vi "UI - Initiate Connection - Copy.vi"(8 "error in (no error)":errorcluster, 10 "Controller Address":string, 11 "Message Queue":refnum<queue>) -> (0 "error out":errorcluster, 1 "Connected?":bool)   [LabVIEW 2017]
uses:
  Message Queue/Message Cluster.ctl
  controls/FPGA State.ctl
  controls/CPU Loads.ctl
  Globals/Global - Configuration Options.vi
  Globals/Global - UI Stream and Variable Connections.vi
  Message Queue/Message Queue.lvlib
panel:
  out "error out 2":errorcluster
  out "tag acc":refnum<k21>
  out "Tag acc":refnum<k21>
  out "Variable Name Control/Indicator 2":refnum<k21>
  out "Variable Name Control/Indicator":refnum<k21>
  out "resulting string 2":string
  out "reader name":string="UI Reader"
  out "writer name":string="UI Writer"
  out "resulting string":string
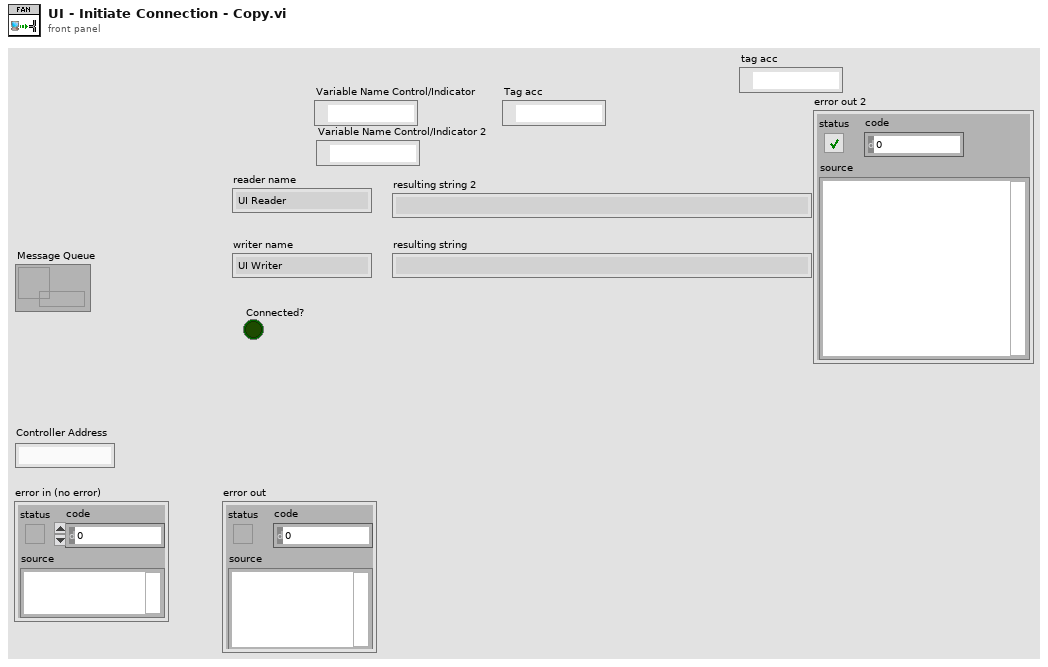
[diagram p1: front panel]
types:
  T1 = typedef "CPU Loads.ctl" = cluster{"Total (%)":dbl, "Time Critical (%)":dbl, "Timed Structures (%)":dbl, "High (%)":dbl, "Above Normal (%)":dbl, "Normal (%)":dbl, "Background (%)":dbl, "Idle (%)":dbl, "ISR (%)":dbl}[]
  T2 = typedef "FPGA State.ctl" = enum16{"Safe State", "Control (PID)"}
  T3 = typedef "Message Queue.lvlib/Message Cluster.ctl" = cluster{"Message":string, "Message Data":variant}
  T4 = cluster{"Actual PID Loop Period":refnum<k21>, "DMA FIFO Overflow?":refnum<k21>, "CPU Usage":refnum<k21>, "Free or Contiguous Memory":refnum<k21>, "Current FPGA State":refnum<k21>, "Acceleration (grms)":refnum<k21>, "Acceleration Waveform":refnum<k21>, "Chatter":refnum<k21>, "tag acc":refnum<k21>, "tag video":refnum<k21>}
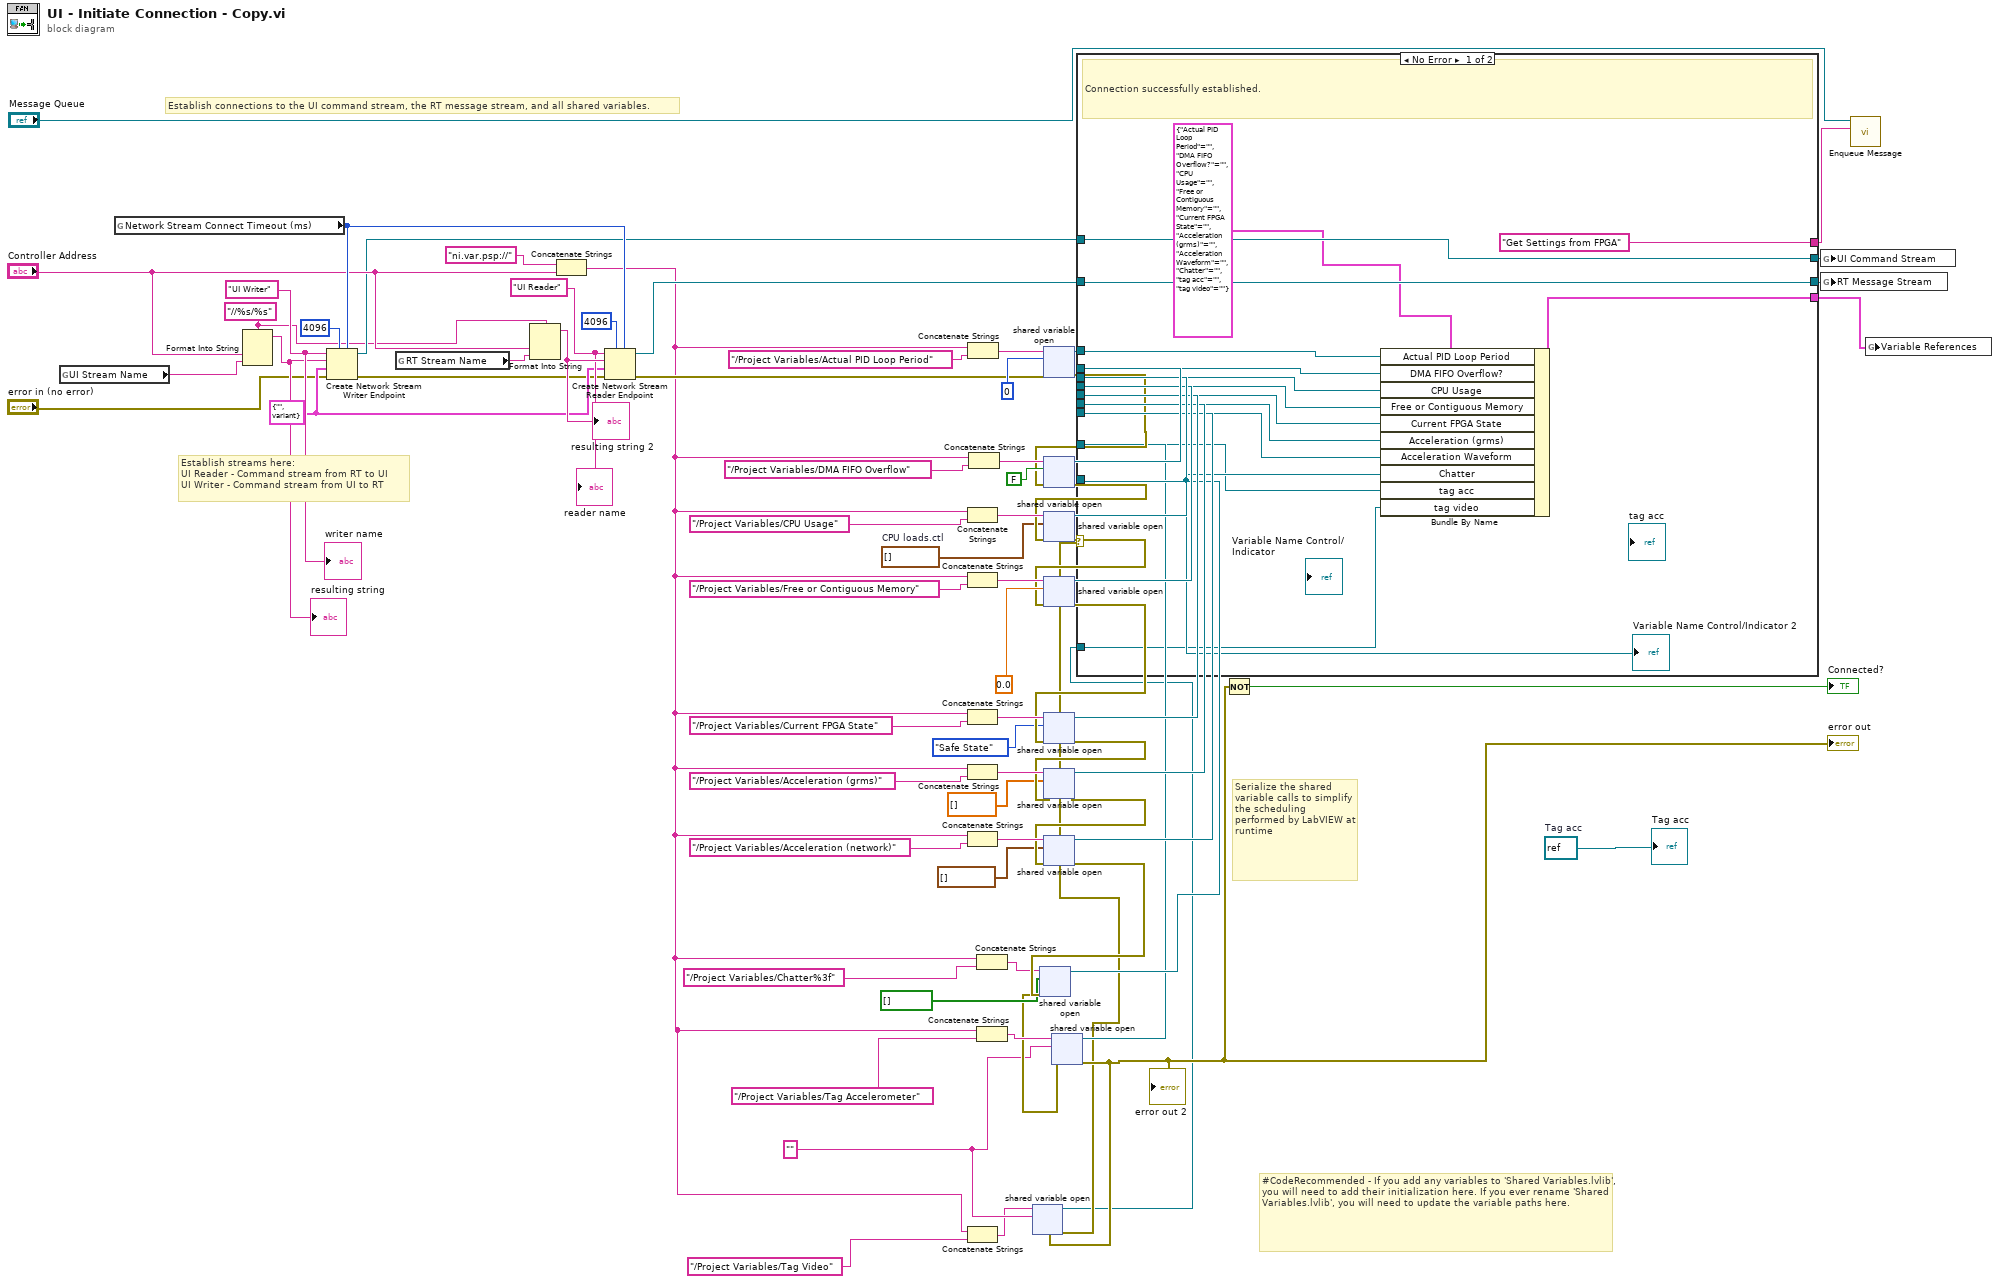
[diagram p0: block diagram]
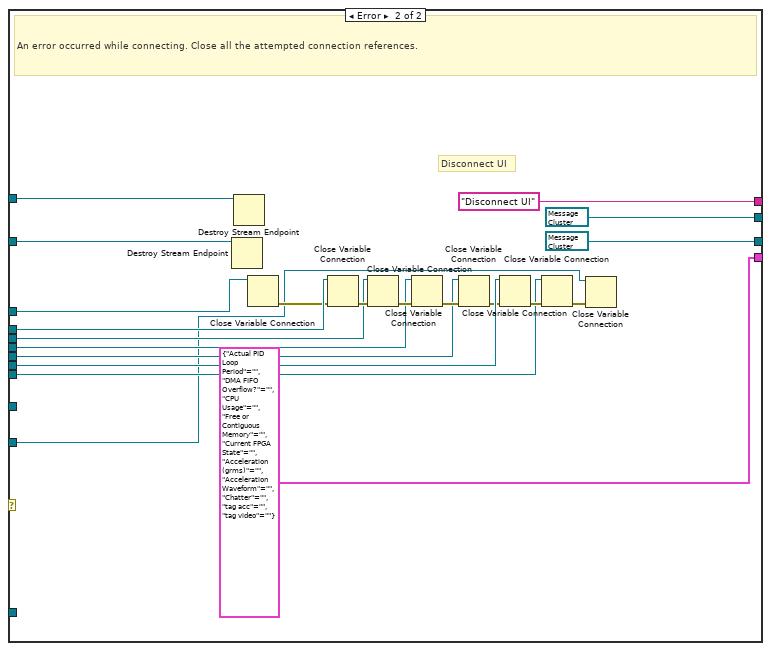
[diagram p2: hidden frame]
diagram:
  w5 = "" ("string")
  w9 = refnum<k21> refnum  # Tag acc
  w24 = T1 []  # CPU loads.ctl
  w70 = T3 {"Message"="", "Message Data"=variant} ("Message Cluster")
  w71 = "UI Reader" ("reader name")
  w74 = "UI Writer" ("writer name")
  w16 = "//%s/%s"
  # "Establish connections to the UI command stream, the RT message stream, and all shared variables."
  # "#CodeRecommended - If you add any variables to 'Shared Variables.lvlib', you will need to add their initialization here. If you ever rename 'Shared Variables.lvlib', you will need to update the variable paths here."
  # "Establish streams here:\nUI Reader - Command stream from RT to UI\nUI Writer - Command stream from UI to RT"
  # "Serialize the shared variable calls to simplify the scheduling performed by LabVIEW at runtime"
  n1 = global read "Global - Configuration Options.vi" "UI Stream Name"() -> (w15:string)
  n2 = global read "Global - Configuration Options.vi" "Network Stream Connect Timeout (ms)"() -> (w69:i32)
  n3 = Format Into String(format string=w16, "Controller Address", w15) -> (resulting string=w73:string)  [unwired: 2 in, 1 out]
  "resulting string" <- w73
  n4 = Create Network Stream Writer Endpoint(5:w69, 7:4096 ("writer buffer size"), 8:"error in (no error)", 9:w70, 10:w73, 11:w74) -> (0:w48:errorcluster, 3:w55:refnum<k21>)  [unwired: 1 in]
  n5 = global read "Global - Configuration Options.vi" "RT Stream Name"() -> (w14:string)
  n6 = Format Into String(format string=w16, "Controller Address", w14) -> (resulting string=w72:string)  [unwired: 2 in, 1 out]
  "resulting string 2" <- w72
  n7 = Concatenate Strings("ni.var.psp://", "Controller Address") -> (w6:string)
  n8 = Create Network Stream Reader Endpoint(5:w69, 7:4096 ("reader buffer size"), 8:w48, 9:w70, 10:w72, 11:w71) -> (0:w47:errorcluster, 3:w54:refnum<k21>)  [unwired: 1 in]
  n9 = Concatenate Strings(w6, "/Project Variables/CPU Usage") -> (w60:string)
  n10 = Concatenate Strings(w6, "/Project Variables/Free or Contiguous Memory") -> (w43:string)
  n11 = Concatenate Strings(w6, "/Project Variables/Current FPGA State") -> (w40:string)
  n12 = Concatenate Strings(w6, "/Project Variables/Acceleration (grms)") -> (w39:string)
  n13 = Concatenate Strings(w6, "/Project Variables/Acceleration (network)") -> (w36:string)
  n14 = Concatenate Strings(w6, "/Project Variables/Tag Video") -> (w1:string)
  n15 = Concatenate Strings(w6, "/Project Variables/Actual PID Loop Period") -> (w65:string)
  n16 = Concatenate Strings(w6, "/Project Variables/DMA FIFO Overflow") -> (w63:string)
  n17 = Concatenate Strings(w6, "/Project Variables/Chatter%3f") -> (w19:string)
  n18 = Concatenate Strings(w6, "/Project Variables/Tag Accelerometer") -> (w13:string)
  n19 = shared-variable-open(w65, w47, u32 0) -> (w58:refnum<k21>, w17:errorcluster)  [unwired: 1 in]
  n20 = shared-variable-open(w63, w17, FALSE ("data type")) -> (w57:refnum<k21>, w59:errorcluster)  [unwired: 1 in]
  n21 = shared-variable-open(w60, w59, w24) -> (w56:refnum<k21>, w35:errorcluster)  [unwired: 1 in]
  n22 = shared-variable-open(w43, w35, 0.0) -> (w30:refnum<k21>, w34:errorcluster)  [unwired: 1 in]
  n23 = shared-variable-open(w40, w34, FPGA_State."Safe State" ("FPGA State")) -> (w29:refnum<k21>, w33:errorcluster)  [unwired: 1 in]
  n24 = shared-variable-open(w39, w33, dbl[] []) -> (w28:refnum<k21>, w32:errorcluster)  [unwired: 1 in]
  n25 = shared-variable-open(w36, w32, waveform(dbl)[] []) -> (w27:refnum<k21>, w21:errorcluster)  [unwired: 1 in]
  n26 = shared-variable-open(w19, w21, bool[] []) -> (w18:refnum<k21>, w10:errorcluster)  [unwired: 1 in]
  n27 = shared-variable-open(w13, w10, w5) -> (w11:refnum<k21>, w4:errorcluster)  [unwired: 1 in]
  "error out" <- w4
  "error out 2" <- w4
  n28 = shared-variable-open(w1, w4, w5) -> (w2:refnum<k21>, w3:errorcluster)  [unwired: 1 in]
  n29 = case shown="No Error" w3 {
    tunnel: w58 -> [w90 w108]
    tunnel: w57 -> [w86 w106]
    tunnel: w56 -> [w85 w107]
    tunnel: w55 -> [w87 w110]
    tunnel: w54 -> [w89 w111]
    tunnel: [w89 refnum<k21> refnum] -> w53
    tunnel: [w87 refnum<k21> refnum] -> w52
    tunnel: ["Get Settings from FPGA" "Disconnect UI"] -> w50
    tunnel: w30 -> [w84 w100]
    tunnel: w29 -> [w83 w99]
    tunnel: w28 -> [w82 w98]
    tunnel: w27 -> [w81 w95]
    tunnel: w18 -> [w80 w92]
    tunnel: w11 -> [w77 _]
    tunnel: [w78 T4 {"Actual PID Loop Period"="", "DMA FIFO Overflow?"="", "CPU Usage"="", "Free or Contiguous Memory"="", "Current FPGA State"="", "Acceleration (grms)"="", "Acceleration Waveform"="", "Chatter"="", "tag acc"="", "tag video"=""} ("Variable References")] -> w8
    tunnel: w2 -> [w76 _]
    frame No Error {
      # "Connection successfully established."
      n30 = Bundle By Name(cluster=T4 {"Actual PID Loop Period"="", "DMA FIFO Overflow?"="", "CPU Usage"="", "Free or Contiguous Memory"="", "Current FPGA State"="", "Acceleration (grms)"="", "Acceleration Waveform"="", "Chatter"="", "tag acc"="", "tag video"=""} ("Variable References"), "Actual PID Loop Period"=w90, "DMA FIFO Overflow?"=w86, "CPU Usage"=w85, "Free or Contiguous Memory"=w84, "Current FPGA State"=w83, "Acceleration (grms)"=w82, "Acceleration Waveform"=w81, "Chatter"=w80, "tag acc"=w77, "tag video"=w76) -> (w78:T4)
      "Variable Name Control/Indicator 2" <- w80
    }
    frame Error {
      # "Disconnect UI"
      # "An error occurred while connecting. Close all the attempted connection references."
      n31 = Destroy Stream Endpoint(11:w111) -> ()  [unwired: 1 in, 1 out]
      n32 = Destroy Stream Endpoint(11:w110) -> ()  [unwired: 1 in, 1 out]
      n33 = Close Variable Connection(11:w108) -> (0:w94:errorcluster)  [unwired: 1 in]
      n34 = Close Variable Connection(8:w94, 11:w106) -> (0:w109:errorcluster)
      n35 = Close Variable Connection(8:w109, 11:w107) -> (0:w102:errorcluster)
      n36 = Close Variable Connection(8:w102, 11:w100) -> (0:w101:errorcluster)
      n37 = Close Variable Connection(8:w101, 11:w99) -> (0:w97:errorcluster)
      n38 = Close Variable Connection(8:w97, 11:w98) -> (0:w96:errorcluster)
      n39 = Close Variable Connection(8:w96, 11:w95) -> (0:w93:errorcluster)
      n40 = Close Variable Connection(8:w93, 11:w92) -> ()  [unwired: 1 out]
    }
  }
  n41 = Not(x=w4) -> (.not. x?=→"Connected?":bool)
  n42 = global write "Global - UI Stream and Variable Connections.vi" "UI Command Stream"(w52) -> ()
  n43 = global write "Global - UI Stream and Variable Connections.vi" "RT Message Stream"(w53) -> ()
  n44 = call "Enqueue Message.vi"("Message"=w50, "Message Queue"="Message Queue") -> ()  [unwired: 8 in, 2 out]
  n45 = global write "Global - UI Stream and Variable Connections.vi" "Variable References"(w8) -> ()
  "writer name" <- w74
  "reader name" <- w71
  "Tag acc" <- w9
